vi "Compile Auto Path.vi"(9 "Scale Right?":bool, 10 "Switch Right?":bool, 11 "Start Left?":bool) -> (3 "Auto Paths":path[](array[path]))   [LabVIEW 2017]
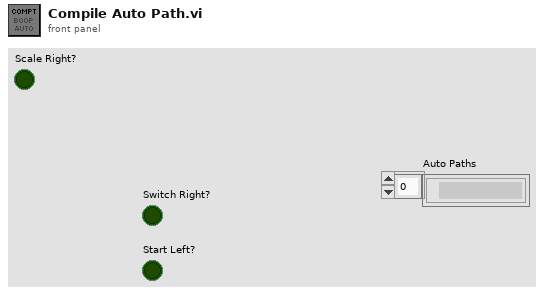
[diagram p1: front panel]
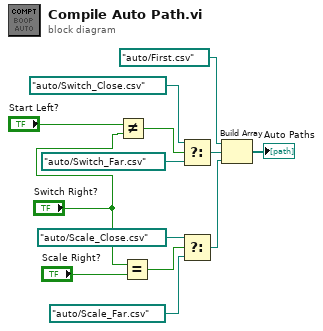
[diagram p0: block diagram]
diagram:
  n1 = Not Equal?(x="Start Left?", y="Switch Right?") -> (x != y?=w3:bool)
  n2 = Equal?(x="Switch Right?", y="Scale Right?") -> (x = y?=w10:bool)
  n3 = Select(t=path "/auto/Switch_Close.csv", s=w3, f=path "/auto/Switch_Far.csv") -> (s? t:f=w5:path)
  n4 = Select(t=path "/auto/Scale_Close.csv", s=w10, f=path "/auto/Scale_Far.csv") -> (s? t:f=w4:path)
  n5 = Build Array(path "/auto/First.csv", w5, w4) -> (→"Auto Paths":path[])
